vi "Main.vi"() -> ()   [LabVIEW 2012]
uses:
  <vilib>/addons/database/Auxilliary.llb/DB Tools Cursor Type.ctl
  <vilib>/Platform/TimedLoop/XDataNode/timing_clust.ctl
  <vilib>/Platform/TimedLoop/XDataNode/nitl_modes.ctl
  <vilib>/Platform/TimedLoop/XDataNode/wakeup.ctl
  <vilib>/addons/database/Connection.llb/DB Tools Open Connec (Path).vi
  <vilib>/addons/database/Connection.llb/Conn Execute.vi
  <vilib>/addons/database/Recordset.llb/Rec Fetch Recordset Data (R).vi
  <vilib>/addons/database/Recordset.llb/Rec Destroy - Connection.vi
  <vilib>/addons/database/Recordset.llb/Rec Get Recordset Properties (R).vi
  <vilib>/addons/database/Recordset.llb/Rec Fetch String Data (R).vi
  <vilib>/addons/database/_DB Variant To Data/Database Variant To Data.xnode
  <vilib>/platform/TimedLoop/XDataNode/XDataNode.xnode
  <vilib>/addons/database/NI_Database_API.lvlib
  <vilib>/Platform/TimedLoop/XDataNode/XDNodeRunTimeDep.lvlib
  GMLibrary.lvlibp
panel:
  in  "ALERTA":bool
  out "Hora / Fecha":timestamp format="%<%X\n%x>T"
  in  "REPORTES":bool
  in  "TRAZAR RUTA":bool
  in  "NUEVO POC":bool
  out "Eventos":string[][](array[string])
  in  "PROGRAMAR":bool
  in  "WebBrowser":refnum<k7>(container)
  in  "stop":bool
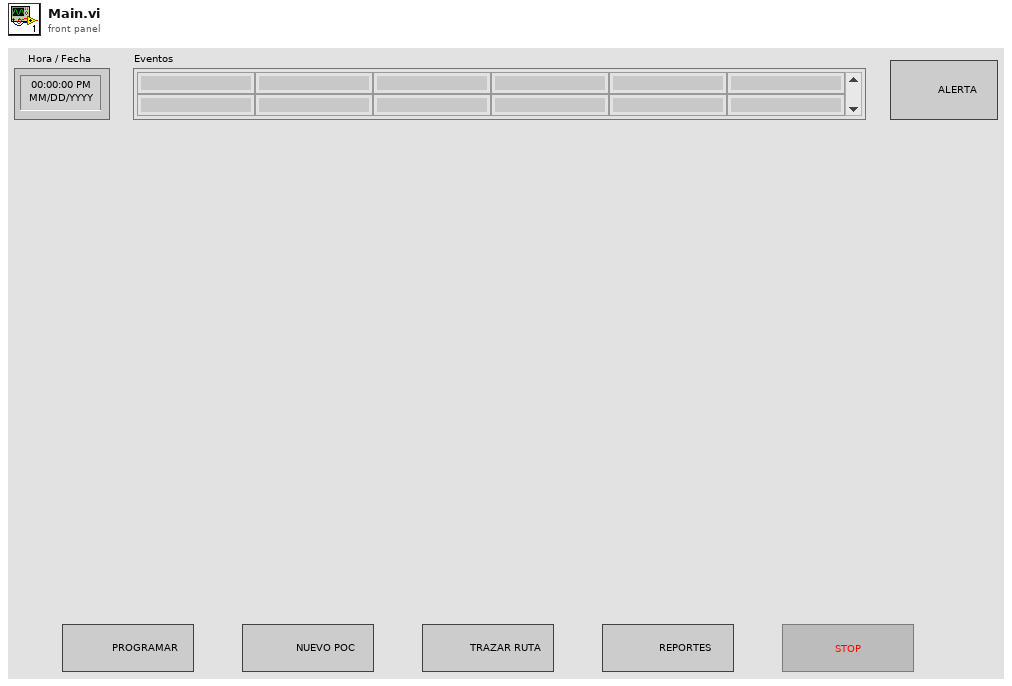
[diagram p1: front panel]
types:
  T1 = typedef "NI_Database_API.lvlib/DB Tools Cursor Type.ctl" = enum16{"forward-only", "keyset", "dynamic", "static"}
  T2 = typedef "NI_Database_API.lvlib/Conn ObjectReference.ctl" = refnum<k1>
  T3 = enum16{"Imei", "POC", "Evento", "Lat", "Lon", "F_H_eve", "F_H_rec", "AVL_N", "AVL_pass", "Propietario", "Razon_Social", "Direccion", "Propietario_N", "Ciudad", "Marca", "Ruta", "N_Ruta", "Auditor", "Auditor_N", "Icon"}
  T4 = enum16{"POC", "Imei", "Evento", "Lat", "Lon", "F_H_eve", "F_H_rec", "AVL_N", "AVL_pass", "Propietario", "Razon_Social", "Direccion", "Propietario_N", "Ciudad", "Marca", "Ruta", "N_Ruta", "Auditor", "Auditor_N"}
  T5 = typedef "NI_Database_API.lvlib/Rec ObjectReference.ctl" = refnum<k1>
  T6 = typedef "XDNodeRunTimeDep.lvlib/timing_clust.ctl" = cluster{"Expected End [f-1]":u64, "Actual End [f-1]":u64, "Finished Late? [f-1]":bool, "Expected End [i-1]":u64, "Actual End [i-1]":u64, "Finished Late? [i-1]":bool, "Expected Start [i]":u64, "Actual Start [i]":u64, "Expected Start [f]":u64, "Actual Start [f]":u64, "Source Name":string, "Structure Name":string, "Period":i64, "Deadline":i64, "Offset":i64, "Start":i64, "Priority":i32, "Timeout":i32, "Mode":T7, "Wakeup Reason":T8, "Error":errorcluster, "Source Type":string, "Secondary Source Type":string, "Global End Time":u64, "Global Start Time":u64, "Frame Duration":u64, "Iteration Duration":u64, "Assigned CPU":i32, "I/O Scan Engine Mode":u32}
  T7 = typedef "XDNodeRunTimeDep.lvlib/nitl_modes.ctl" = enum32{"No Change", "Process missed periods, maintain original phase", "Discard missed periods, maintain original phase", "Process missed periods, ignore original phase", "Discard missed periods, ignore original phase"}
  T8 = typedef "XDNodeRunTimeDep.lvlib/wakeup.ctl" = enum32{"Normal", "Aborted", "Asynchronous wakeup", "Timing source error", "Timed loop error", "Timeout"}
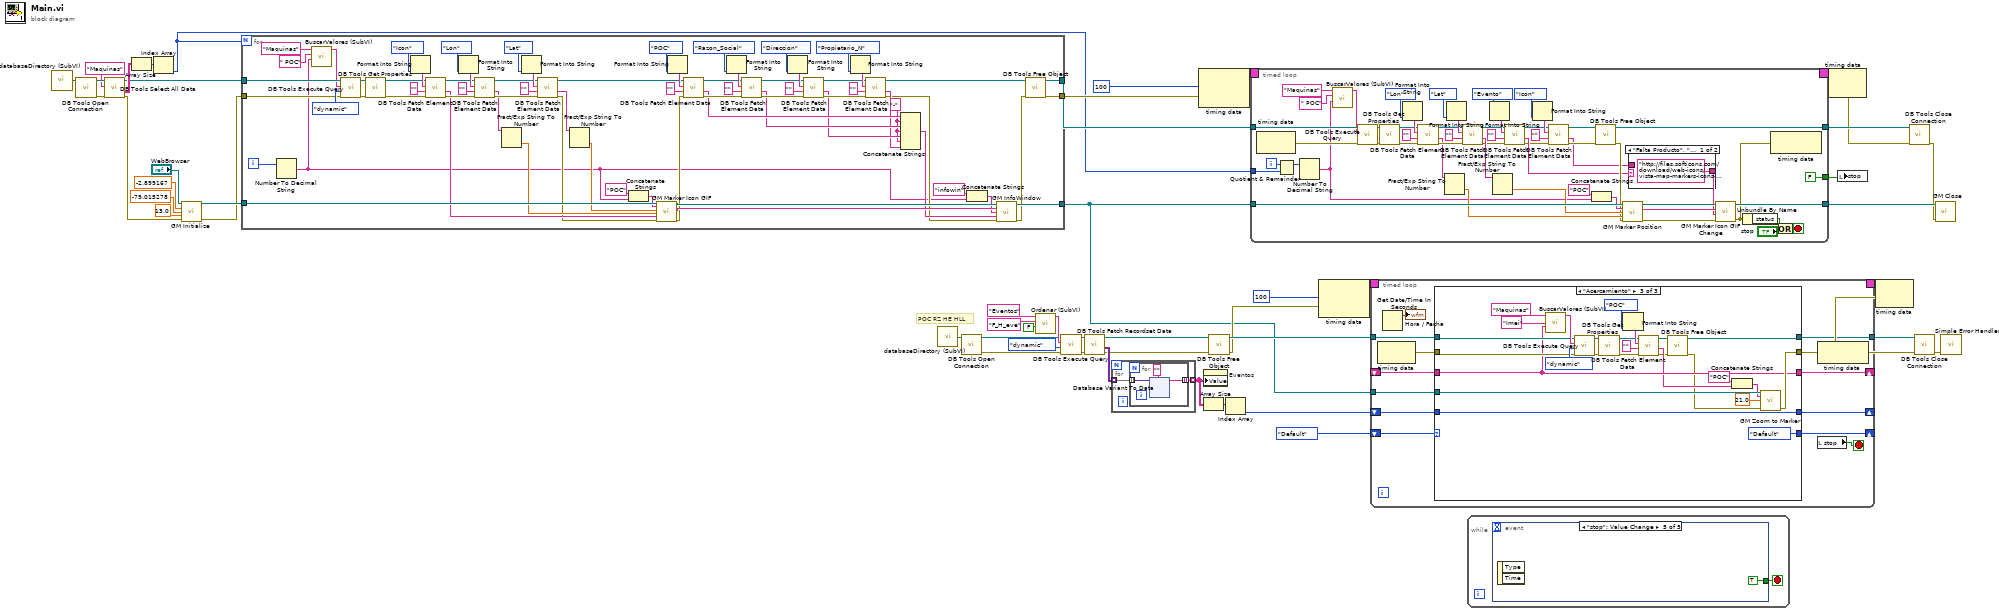
[diagram p0: block diagram]
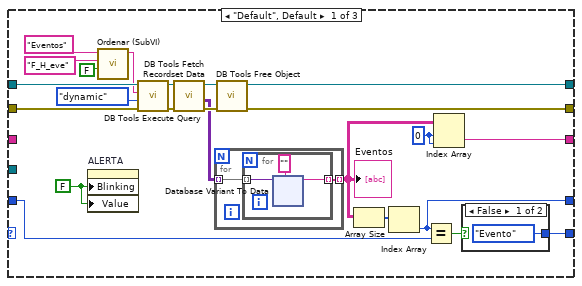
[diagram p2: hidden frame]
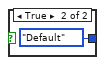
[diagram p3: hidden frame]
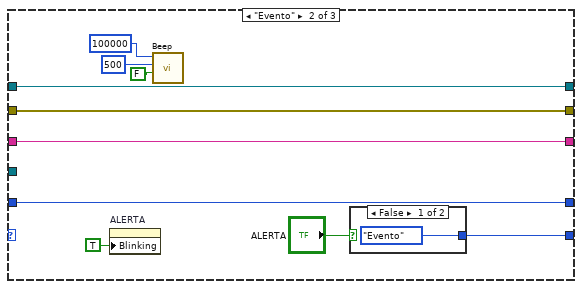
[diagram p4: hidden frame]
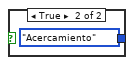
[diagram p5: hidden frame]
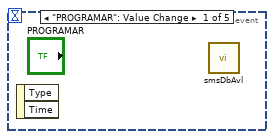
[diagram p6: hidden frame]
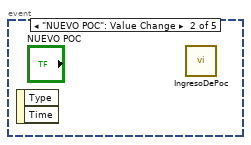
[diagram p7: hidden frame]
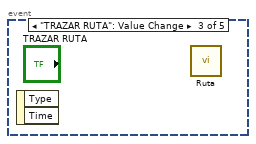
[diagram p8: hidden frame]
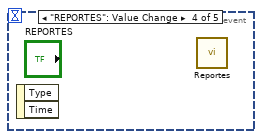
[diagram p9: hidden frame]
diagram:
  # "POC RZ HE HLL"
  n1 = call "databaseDirectory (SubVI).vi"() -> ("Application Directory"=w29:path)  [unwired: 1 in]
  n2 = call-poly <vilib>:"DB Tools Open Connection.vi"("connection information"=w29) -> ("error out"=w49:errorcluster, "connection reference"=w48:T2)  [unwired: 7 in]
  n3 = call <vilib>:"DB Tools Select All Data.vi"("error in (no error)"=w49, "table"="Maquinas", "connection reference"=w48) -> ("error out"=w39:errorcluster, "data"=w51:string[][], "connection reference out"=w47:T2)  [unwired: 3 in]
  n4 = Array Size(array=w51) -> (size(s)=w50:i32[])
  n5 = Index Array(array=w50) -> (element=w30:i32)  [unwired: 1 in]
  n6 = call "GM Initialize.vi"("Automation Refnum in"="WebBrowser", "Latitude"=-2.899167, "Longitude"=-79.015278, "Zoom"=13.0, "Error In"=w39) -> ("Automation Refnum out"=w42:refnum<k7>, "Error Out"=w38:errorcluster)  [unwired: 8 in, 1 out]
  n7 = for {
    N: w30 -> [_]
    tunnel: w47 -> [w114]
    tunnel: w38 -> [w115]
    tunnel: w42 -> [w111]
    tunnel: [w98] -> w2
    tunnel: [w95] -> w35
    tunnel: [w57] -> w36
    i -> [w52]
    w71 = "-" ("type")
    n8 = Number To Decimal String(number=w52) -> (decimal integer string=w56:string)  [unwired: 1 in]
    n9 = call "BuscarValores (SubVI).vi"("="=w56, "Columna"=" POC" ("Substring"), "Tabla"="Maquinas" ("table")) -> ("String"=w55:string)  [unwired: 8 in]
    n10 = call-poly <vilib>:"DB Tools Execute Query.vi"("error in (no error)"=w115, "cursor type"=DB_Tools_Cursor_Type."dynamic", "SQL query"=w55, "connection reference"=w114) -> ("error out"=w117:errorcluster, "recordset reference"=w118:T5)  [unwired: 4 in]
    n11 = call-poly <vilib>:"DB Tools Get Properties.vi"("error in (no error)"=w117, "recordset reference"=w118) -> ("error out"=w65:errorcluster, "recordset reference out"=w66:T5)  [unwired: 3 in, 1 out]
    n12 = Format Into String(T3."Icon") -> (resulting string=w67:string)  [unwired: 3 in, 1 out]
    n13 = call-poly <vilib>:"DB Tools Fetch Element Data.vi"("error in (no error)"=w65, "type"="", "column index"=w67, "recordset reference"=w66) -> ("error out"=w63:errorcluster, "data"=w62:string, "recordset reference out"=w64:T5)  [unwired: 3 in]
    n14 = Format Into String(T4."Lon") -> (resulting string=w121:string)  [unwired: 3 in, 1 out]
    n15 = call-poly <vilib>:"DB Tools Fetch Element Data.vi"("error in (no error)"=w63, "type"="", "column index"=w121, "recordset reference"=w64) -> ("error out"=w103:errorcluster, "data"=w102:string, "recordset reference out"=w104:T5)  [unwired: 3 in]
    n16 = Fract/Exp String To Number(string=w102) -> (number=w99:dbl)  [unwired: 3 in, 1 out]
    n17 = Format Into String(T4."Lat") -> (resulting string=w105:string)  [unwired: 3 in, 1 out]
    n18 = call-poly <vilib>:"DB Tools Fetch Element Data.vi"("error in (no error)"=w103, "type"="", "column index"=w105, "recordset reference"=w104) -> ("error out"=w61:errorcluster, "data"=w101:string, "recordset reference out"=w92:T5)  [unwired: 3 in]
    n19 = Fract/Exp String To Number(string=w101) -> (number=w100:dbl)  [unwired: 3 in, 1 out]
    n20 = Concatenate Strings("POC" ("Marker Name"), w56) -> (w110:string)
    n21 = call "GM Marker Icon GIF.vi"("Automation Refnum in"=w111, "Marker Name"=w110, "Latitude"=w100, "Longitude"=w99, "Icon"=w62, "error in (no error)"=w61) -> ("Automation Refnum out"=w113:refnum<k7>, "Marker Name"=w112:string, "error out"=w60:errorcluster)  [unwired: 11 in]
    n22 = Format Into String(T4."POC") -> (resulting string=w93:string)  [unwired: 3 in, 1 out]
    n23 = call-poly <vilib>:"DB Tools Fetch Element Data.vi"("error in (no error)"=w60, "type"="", "column index"=w93, "recordset reference"=w92) -> ("error out"=w88:errorcluster, "data"=w75:string, "recordset reference out"=w89:T5)  [unwired: 3 in]
    n24 = Format Into String(T4."Razon_Social") -> (resulting string=w91:string)  [unwired: 3 in, 1 out]
    n25 = call-poly <vilib>:"DB Tools Fetch Element Data.vi"("error in (no error)"=w88, "type"="", "column index"=w91, "recordset reference"=w89) -> ("error out"=w84:errorcluster, "data"=w74:string, "recordset reference out"=w85:T5)  [unwired: 3 in]
    n26 = Format Into String(T4."Direccion") -> (resulting string=w97:string)  [unwired: 3 in, 1 out]
    n27 = call-poly <vilib>:"DB Tools Fetch Element Data.vi"("error in (no error)"=w84, "type"="", "column index"=w97, "recordset reference"=w85) -> ("error out"=w82:errorcluster, "data"=w73:string, "recordset reference out"=w83:T5)  [unwired: 3 in]
    n28 = Format Into String(T4."Propietario_N") -> (resulting string=w86:string)  [unwired: 3 in, 1 out]
    n29 = call-poly <vilib>:"DB Tools Fetch Element Data.vi"("error in (no error)"=w82, "type"="", "column index"=w86, "recordset reference"=w83) -> ("error out"=w59:errorcluster, "data"=w72:string, "recordset reference out"=w76:T5)  [unwired: 3 in]
    n30 = Concatenate Strings(w75, w71, w74, w71, w73, w71, w72) -> (w70:string)
    n31 = Concatenate Strings("infowin" ("InfoWindow Name"), w56) -> (w107:string)
    n32 = call "GM InfoWindow.vi"("Automation Refnum in"=w113, "Marker Name"=w112, "InfoWindow Name"=w107, "Message"=w70, "error in (no error)"=w59) -> ("Automation Refnum out"=w98:refnum<k7>, "error out"=w58:errorcluster)  [unwired: 9 in]
    n33 = call-poly <vilib>:"DB Tools Free Object.vi"("error in (no error)"=w58, "recordset reference"=w76) -> ("error out"=w57:errorcluster, "connection reference"=w95:T2)  [unwired: 8 in]
  }
  n34 = call "databaseDirectory (SubVI).vi"() -> ("Application Directory"=w26:path)  [unwired: 1 in]
  n35 = call-poly <vilib>:"DB Tools Open Connection.vi"("connection information"=w26) -> ("error out"=w14:errorcluster, "connection reference"=w13:T2)  [unwired: 7 in]
  n36 = call "Ordenar (SubVI).vi"("Orden"=FALSE, "Columna"="F_H_eve", "Tabla"="Eventos") -> ("String"=w18:string)  [unwired: 8 in]
  n37 = call-poly <vilib>:"DB Tools Execute Query.vi"("error in (no error)"=w14, "cursor type"=DB_Tools_Cursor_Type."dynamic", "SQL query"=w18, "connection reference"=w13) -> ("error out"=w17:errorcluster, "recordset reference"=w16:T5)  [unwired: 4 in]
  n38 = call-poly <vilib>:"DB Tools Fetch Recordset Data.vi"("error in (no error)"=w17, "recordset reference"=w16) -> ("error out"=w23:errorcluster, "recordset data"=w24:variant[][], "recordset reference out"=w22:T5)  [unwired: 3 in]
  n39 = for {
    tunnel: w24 -> [w123] mode=indexing
    tunnel: [w122] -> w11 mode=indexing
    n40 = for {
      tunnel: w123 -> [w125] mode=indexing
      tunnel: [w124] -> w122 mode=indexing
      n41 = xnode "Database Variant To Data"("database variant"=w125, "type"="") -> ("data"=w124:string)  [unwired: 1 in, 1 out]
    }
  }
  n42 = node-c288(i64 100 ("Period"), w36) -> (w46:T6)
  n43 = Array Size(array=w11) -> (size(s)=w12:i32[])
  n44 = property on="Eventos" class="Arr (strict)"("Value"=w11) -> ()  [unwired: 2 in, 2 out]
  n45 = call-poly <vilib>:"DB Tools Free Object.vi"("error in (no error)"=w23, "recordset reference"=w22) -> ("error out"=w7:errorcluster, "connection reference"=w15:T2)  [unwired: 8 in]
  n46 = Index Array(array=w12) -> (element=w5:i32)  [unwired: 1 in]
  n47 = timed-loop {
    timing: w46 -> [_]
    timing-out: [_] -> w45
    tunnel: w2 -> [w204]
    tunnel: w35 -> [w207]
    tunnel: [w171] -> w34
    tunnel: [w199] -> w33
    tunnel: w30 -> [w198]
    tunnel: [FALSE ("stop")] -> w1
    i -> [w205]
    stop <- w211 stop-if-true
    n48 = node-c288() -> (w206:errorcluster)  [unwired: 1 in]
    n49 = Quotient & Remainder(x=w205, y=w198) -> (x-y*floor(x/y)=w181:i32)  [unwired: 1 out]
    n50 = Number To Decimal String(number=w181) -> (decimal integer string=w195:string)  [unwired: 1 in]
    n51 = call "BuscarValores (SubVI).vi"("="=w195, "Columna"=" POC" ("Substring"), "Tabla"="Maquinas" ("table")) -> ("String"=w194:string)  [unwired: 8 in]
    n52 = call-poly <vilib>:"DB Tools Execute Query.vi"("error in (no error)"=w206, "SQL query"=w194, "connection reference"=w207) -> ("error out"=w208:errorcluster, "recordset reference"=w209:T5)  [unwired: 5 in]
    n53 = call-poly <vilib>:"DB Tools Get Properties.vi"("error in (no error)"=w208, "recordset reference"=w209) -> ("error out"=w184:errorcluster, "recordset reference out"=w185:T5)  [unwired: 3 in, 1 out]
    n54 = Format Into String(T4."Lon") -> (resulting string=w193:string)  [unwired: 3 in, 1 out]
    n55 = call-poly <vilib>:"DB Tools Fetch Element Data.vi"("error in (no error)"=w184, "type"="", "column index"=w193, "recordset reference"=w185) -> ("error out"=w187:errorcluster, "data"=w182:string, "recordset reference out"=w188:T5)  [unwired: 3 in]
    n56 = Fract/Exp String To Number(string=w182) -> (number=w202:dbl)  [unwired: 3 in, 1 out]
    n57 = Format Into String(T4."Lat") -> (resulting string=w189:string)  [unwired: 3 in, 1 out]
    n58 = call-poly <vilib>:"DB Tools Fetch Element Data.vi"("error in (no error)"=w187, "type"="", "column index"=w189, "recordset reference"=w188) -> ("error out"=w176:errorcluster, "data"=w183:string, "recordset reference out"=w177:T5)  [unwired: 3 in]
    n59 = Format Into String(T4."Evento") -> (resulting string=w179:string)  [unwired: 3 in, 1 out]
    n60 = Fract/Exp String To Number(string=w183) -> (number=w203:dbl)  [unwired: 3 in, 1 out]
    n61 = call-poly <vilib>:"DB Tools Fetch Element Data.vi"("error in (no error)"=w176, "type"="", "column index"=w179, "recordset reference"=w177) -> ("error out"=w165:errorcluster, "data"=w169:string, "recordset reference out"=w166:T5)  [unwired: 3 in]
    n62 = Format Into String(T3."Icon") -> (resulting string=w167:string)  [unwired: 3 in, 1 out]
    n63 = call-poly <vilib>:"DB Tools Fetch Element Data.vi"("error in (no error)"=w165, "type"="", "column index"=w167, "recordset reference"=w166) -> ("error out"=w162:errorcluster, "data"=w161:string, "recordset reference out"=w163:T5)  [unwired: 3 in]
    n64 = Concatenate Strings("POC" ("Marker Name"), w195) -> (w200:string)
    n65 = call-poly <vilib>:"DB Tools Free Object.vi"("error in (no error)"=w162, "recordset reference"=w163) -> ("error out"=w175:errorcluster, "connection reference"=w199:T2)  [unwired: 8 in]
    n66 = call "GM Marker Position.vi"("Automation Refnum in"=w204, "Marker Name"=w200, "Latitude"=w203, "Longitude"=w202, "error in (no error)"=w175) -> ("Automation Refnum out"=w174:refnum<k7>, "Marker Name"=w172:string, "error out"=w173:errorcluster)  [unwired: 8 in]
    n67 = case shown="\"Falta Producto\", \"Máquina Abierta\", \"Servicio Técnico\"" w169 {
      tunnel: ["http://files.softicons.com/download/web-icons/vista-map-markers-icons-by-icons-land/png/128x128/MapMarker_PushPin2_Left_Pink.png" ("data") w214] -> w168
      tunnel: w161 -> [_ w214]
      frame "Falta Producto", "Máquina Abierta", "Servicio Técnico" {
      }
      frame "Automático", Default {
      }
    }
    n68 = call "GM Marker Icon GIF Change.vi"("error in (no error)"=w173, "Icon"=w168, "Marker Name"=w172, "Automation Refnum in"=w174) -> ("error out"=w170:errorcluster, "Automation Refnum out"=w171:refnum<k7>)  [unwired: 1 out]
    n69 = Unbundle By Name(w170) -> ("status"=w212:bool)
    n70 = node-c288(w170) -> ()  [unwired: 1 out]
    n71 = Or(x=w212, y="stop") -> (x .or. y?=w211:bool)
  }
  n72 = node-c288(i64 100 ("Period"), w7) -> (w10:T6)
  n73 = timed-loop {
    tunnel: w15 -> [w232]
    tunnel: [w231] -> w27
    timing: w10 -> [_]
    timing-out: [_] -> w9
    shift-right: [w227] -> _
    shift-left: enum16{"Default", "Evento", "Acercamiento"}."Default" -> [w226]
    shift-right: [w224] -> _
    shift-left: w5 -> [w225]
    shift-right: [w222] -> _
    shift-left: _ -> [w221]
    tunnel: w2 -> [w220]
    stop <- w223 stop-if-true
    n74 = node-c288() -> (w230:errorcluster)  [unwired: 1 in]
    n75 = Get Date/Time In Seconds() -> (seconds since 1Jan1904=→"Hora / Fecha":timestamp)
    n76 = case shown="\"Acercamiento\"" w226 {
      tunnel: w232 -> [w255 w304 w319]
      tunnel: [w254 w304 w307] -> w231
      tunnel: w230 -> [w253 w303 w318]
      tunnel: [w252 w303 w313] -> w229
      tunnel: [w236 w296 enum16{"Default", "Evento", "Acercamiento"}."Default"] -> w227
      tunnel: w225 -> [w240 w302 w331]
      tunnel: [w239 w302 w331] -> w224
      tunnel: [w233 w295 w312] -> w222
      tunnel: w221 -> [_ w295 w312]
      tunnel: w220 -> [_ _ w316]
      frame "Default", Default {
        w234 = 0 ("index (row)")
        w238 = FALSE ("Blinking")
        n77 = property on="ALERTA" class="Bool (strict)"("Blinking"=w238, "Value"=w238) -> ()  [unwired: 2 in, 2 out]
        n78 = call "Ordenar (SubVI).vi"("Orden"=FALSE, "Columna"="F_H_eve", "Tabla"="Eventos") -> ("String"=w249:string)  [unwired: 8 in]
        n79 = call-poly <vilib>:"DB Tools Execute Query.vi"("error in (no error)"=w253, "cursor type"=DB_Tools_Cursor_Type."dynamic", "SQL query"=w249, "connection reference"=w255) -> ("error out"=w250:errorcluster, "recordset reference"=w251:T5)  [unwired: 4 in]
        n80 = call-poly <vilib>:"DB Tools Fetch Recordset Data.vi"("error in (no error)"=w250, "recordset reference"=w251) -> ("error out"=w244:errorcluster, "recordset data"=w243:variant[][], "recordset reference out"=w245:T5)  [unwired: 3 in]
        n81 = for {
          tunnel: w243 -> [w259] mode=indexing
          tunnel: [w258] -> w235 mode=indexing
          n82 = for {
            tunnel: w259 -> [w261] mode=indexing
            tunnel: [w260] -> w258 mode=indexing
            n83 = xnode "Database Variant To Data"("database variant"=w261, "type"="") -> ("data"=w260:string)  [unwired: 1 in, 1 out]
          }
        }
        "Eventos" <- w235
        n84 = call-poly <vilib>:"DB Tools Free Object.vi"("error in (no error)"=w244, "recordset reference"=w245) -> ("error out"=w252:errorcluster, "connection reference"=w254:T2)  [unwired: 8 in]
        n85 = Array Size(array=w235) -> (size(s)=w241:i32[])
        n86 = Index Array(array=w241) -> (element=w239:i32)  [unwired: 1 in]
        n87 = Equal?(x=w239, y=w240) -> (x = y?=w237:bool)
        n88 = Index Array(array=w235, index (row)=w234, index (col)=w234) -> (element=w233:string)
        n89 = case shown="False" w237 {
          tunnel: [enum16{"Default", "Evento", "Acercamiento"}."Evento" enum16{"Default", "Evento", "Acercamiento"}."Default"] -> w236
          frame False {
          }
          frame True {
          }
        }
      }
      frame "Evento" {
        n90 = property on="ALERTA" class="Bool (strict)"("Blinking"=TRUE) -> ()  [unwired: 2 in, 2 out]
        n91 = call <vilib>:"Beep.vi"("use system alert? (T)"=FALSE, "duration (msec)"=u32 500, "frequency (Hz)"=u32 100000) -> ()  [unwired: 9 in]
        n92 = case shown="False" "ALERTA" {
          tunnel: [enum16{"Default", "Evento", "Acercamiento"}."Evento" enum16{"Default", "Evento", "Acercamiento"}."Acercamiento"] -> w296
          frame False {
          }
          frame True {
          }
        }
      }
      frame "Acercamiento" {
        n93 = call "BuscarValores (SubVI).vi"("="=w312, "Columna"="Imei", "Tabla"="Maquinas") -> ("String"=w330:string)  [unwired: 8 in]
        n94 = call-poly <vilib>:"DB Tools Execute Query.vi"("error in (no error)"=w318, "cursor type"=DB_Tools_Cursor_Type."dynamic", "SQL query"=w330, "connection reference"=w319) -> ("error out"=w327:errorcluster, "recordset reference"=w328:T5)  [unwired: 4 in]
        n95 = call-poly <vilib>:"DB Tools Get Properties.vi"("error in (no error)"=w327, "recordset reference"=w328) -> ("error out"=w322:errorcluster, "recordset reference out"=w323:T5)  [unwired: 3 in, 1 out]
        n96 = Format Into String(T3."POC") -> (resulting string=w324:string)  [unwired: 3 in, 1 out]
        n97 = call-poly <vilib>:"DB Tools Fetch Element Data.vi"("error in (no error)"=w322, "type"="", "column index"=w324, "recordset reference"=w323) -> ("error out"=w309:errorcluster, "data"=w311:string, "recordset reference out"=w310:T5)  [unwired: 3 in]
        n98 = call-poly <vilib>:"DB Tools Free Object.vi"("error in (no error)"=w309, "recordset reference"=w310) -> ("error out"=w308:errorcluster, "connection reference"=w307:T2)  [unwired: 8 in]
        n99 = Concatenate Strings("POC" ("Marker Name"), w311) -> (w314:string)
        n100 = call "GM Zoom to Marker.vi"("Automation Refnum in"=w316, "Marker Name"=w314, "Zoom"=21.0, "error in (no error)"=w308) -> ("error out"=w313:errorcluster)  [unwired: 9 in, 2 out]
      }
    }
    n101 = node-c288(w229) -> ()  [unwired: 1 out]
    n102 = local read "stop"() -> (w223:bool)
  }
  n103 = while {
    stop <- w338 stop-if-true
    n104 = event shown="[4] \"stop\": Value Change" {
      selector: _ -> [_ _ _ _ _]
      dyn-events: _ -> [_ _ _ _ _]
      timeout: _ -> [_ _ _ _ _]
      tunnel: [_ _ _ _ TRUE] -> w338
      event "PROGRAMAR": Value Change {
        n105 = event-data() -> ()  [unwired: 1 in, 2 out]
        n106 = call "smsDbAvl.vi"() -> ()  [unwired: 12 in]
      }
      event "NUEVO POC": Value Change {
        n107 = event-data() -> ()  [unwired: 1 in, 2 out]
        n108 = call "IngresoDePoc.vi"() -> ()  [unwired: 12 in]
      }
      event "TRAZAR RUTA": Value Change {
        n109 = event-data() -> ()  [unwired: 1 in, 2 out]
        n110 = call "Ruta.vi"() -> ()  [unwired: 12 in]
      }
      event "REPORTES": Value Change {
        n111 = event-data() -> ()  [unwired: 1 in, 2 out]
        n112 = call "Reportes.vi"() -> ()  [unwired: 12 in]
      }
      event "stop": Value Change {
        n113 = event-data() -> ()  [unwired: 1 in, 2 out]
      }
    }
  }
  n114 = node-c288(w45) -> (w32:errorcluster)
  n115 = local write "stop"(w1) -> ()
  n116 = node-c288(w9) -> (w6:errorcluster)
  n117 = call <vilib>:"DB Tools Close Connection.vi"("error in (no error)"=w32, "connection reference"=w33) -> ("error out"=w31:errorcluster)  [unwired: 5 in]
  n118 = call <vilib>:"DB Tools Close Connection.vi"("error in (no error)"=w6, "connection reference"=w27) -> ("error out"=w28:errorcluster)  [unwired: 5 in]
  n119 = call "GM Close.vi"("error in (no error)"=w31, "Automation Refnum in"=w34) -> ()  [unwired: 9 in, 1 out]
  n120 = call <vilib>:"Simple Error Handler.vi"("error in (no error)"=w28) -> ()  [unwired: 4 in, 5 out]
